vi "barometerCal.vi"(2 "Calibration":u16[](array[numeric]) format="%x", 3 "(int16)Pressure":u16 format="%x", 4 "(uint16) Temp":u16 format="%x") -> (0 "Pressure":dbl, 1 "Temperature":dbl)   [LabVIEW 2012]
panel:
  # "C"
  # "Pa"
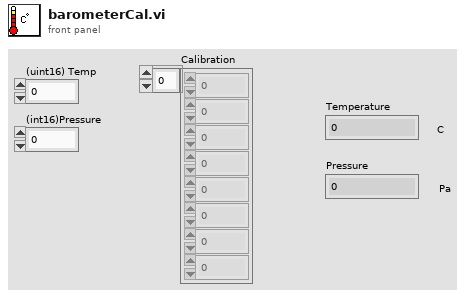
[diagram p1: front panel]
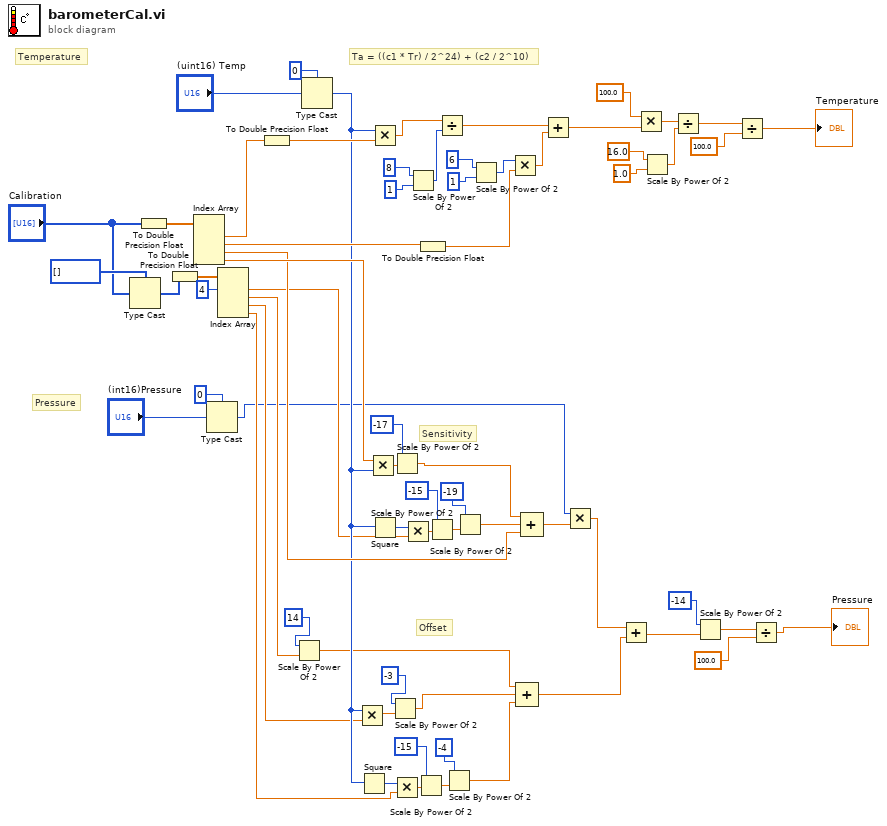
[diagram p0: block diagram]
diagram:
  # "Offset"
  # "Sensitivity"
  # "Pressure"
  # "Temperature"
  # "Ta = ((c1 * Tr) / 2^24) + (c2 / 2^10)"
  n1 = Type Cast(type=i16[] [], x="Calibration") -> (*(type *) &x=w11:i16[])
  n2 = To Double Precision Float(number="Calibration") -> (double precision float=w45:dbl[])
  n3 = To Double Precision Float(number=w11) -> (double precision float=w10:dbl[])
  n4 = Index Array(array=w45) -> (element #1=w55:dbl, element #2=w50:dbl, element #3=w34:dbl, element #4=w43:dbl)  [unwired: 4 in]
  n5 = Type Cast(type=u16 0, x="(int16)Pressure") -> (*(type *) &x=w1:u16)
  n6 = Index Array(array=w10, index #1=4 ("index")) -> (element #1=w16:dbl, element #2=w15:dbl, element #3=w14:dbl, element #4=w13:dbl)  [unwired: 3 in]
  n7 = To Double Precision Float(number=w55) -> (double precision float=w54:dbl)
  n8 = Scale By Power Of 2(n=i16 14, x=w15) -> (x*2^n=w24:dbl)
  n9 = Type Cast(type=i16 0, x="(uint16) Temp") -> (*(type *) &x=w25:i16)
  n10 = Multiply(x=w25, y=w14) -> (x*y=w31:dbl)
  n11 = Square(x=w25) -> (x^2=w28:i16)
  n12 = Multiply(x=w43, y=w25) -> (x*y=w42:dbl)
  n13 = Multiply(x=w25, y=w54) -> (x*y=w65:dbl)
  n14 = Square(x=w25) -> (x^2=w39:i16)
  n15 = Scale By Power Of 2(n=i16 -3, x=w31) -> (x*2^n=w23:dbl)
  n16 = Scale By Power Of 2(n=i16 -17, x=w42) -> (x*2^n=w35:dbl)
  n17 = Multiply(x=w28, y=w13) -> (x*y=w29:dbl)
  n18 = Multiply(x=w39, y=w16) -> (x*y=w40:dbl)
  n19 = Scale By Power Of 2(n=i16 8, x=i16 1) -> (x*2^n=w66:i16)
  n20 = Scale By Power Of 2(n=i16 -15, x=w29) -> (x*2^n=w26:dbl)
  n21 = To Double Precision Float(number=w50) -> (double precision float=w51:dbl)
  n22 = Scale By Power Of 2(n=i16 -15, x=w40) -> (x*2^n=w37:dbl)
  n23 = Divide(x=w65, y=w66) -> (x/y=w52:dbl)
  n24 = Scale By Power Of 2(n=i16 -4, x=w26) -> (x*2^n=w22:dbl)
  n25 = Scale By Power Of 2(n=i16 -19, x=w37) -> (x*2^n=w36:dbl)
  n26 = Scale By Power Of 2(n=i16 6, x=i16 1) -> (x*2^n=w62:i16)
  n27 = Multiply(x=w62, y=w51) -> (x*y=w61:dbl)
  n28 = Compound Arithmetic op=ADD(w24, w23, w22) -> (w18:dbl)
  n29 = Compound Arithmetic op=ADD(w35, w36, w34) -> (w20:dbl)
  n30 = Add(x=w52, y=w61) -> (x+y=w56:dbl)
  n31 = Multiply(x=w1, y=w20) -> (x*y=w19:dbl)
  n32 = Add(x=w19, y=w18) -> (x+y=w17:dbl)
  n33 = Multiply(x=100.0 ("n"), y=w56) -> (x*y=w49:dbl)
  n34 = Scale By Power Of 2(n=16.0, x=1.0) -> (x*2^n=w57:dbl)
  n35 = Divide(x=w49, y=w57) -> (x/y=w48:dbl)
  n36 = Scale By Power Of 2(n=i16 -14, x=w17) -> (x*2^n=w8:dbl)
  n37 = Divide(x=w48, y=100.0 ("n")) -> (x/y=→"Temperature":dbl)
  n38 = Divide(x=w8, y=100.0 ("n")) -> (x/y=→"Pressure":dbl)
